vi "Servo_global.vi"() -> ()   [LabVIEW 2020, in "输出轴伺服.lvlib"]
panel:
  out "AxisHandle":u32
  out "DeviceHandle":u32
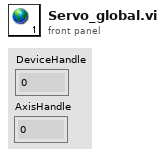
[diagram p1: front panel]
diagram:
